vi "ValueConcat.vi"(9 "Length":dbl, 11 "Value":dbl) -> (2 "Output":string)   [LabVIEW 2010]
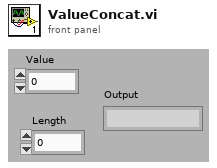
[diagram p1: front panel]
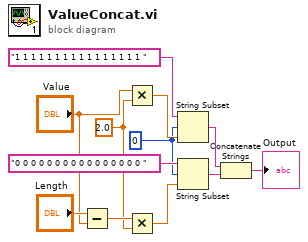
[diagram p0: block diagram]
diagram:
  w5 = 0 ("offset (0)")
  w7 = 2.0 ("y")
  n1 = Subtract(x="Length", y="Value") -> (x-y=w8:dbl)
  n2 = Multiply(x="Value", y=w7) -> (x*y=w11:dbl)
  n3 = Multiply(x=w8, y=w7) -> (x*y=w4:dbl)
  n4 = String Subset(string="1 1 1 1 1 1 1 1 1 1 1 1 1 1 1 1 ", offset (0)=w5, length (rest)=w11) -> (substring=w2:string)
  n5 = String Subset(string="0 0 0 0 0 0 0 0 0 0 0 0 0 0 0 0 ", offset (0)=w5, length (rest)=w4) -> (substring=w3:string)
  n6 = Concatenate Strings(w2, w3) -> (→"Output":string)
